vi "SATDdll.vi"(8 "error in (no error)":errorcluster, 11 "SAT Inputs":cluster{"D":dbl, "z":dbl[], "kph":i32}={"D"=0.0, "z"=[0.0, 0.0, 0.0, 0.0, 0.0, 0.0, 0.0, 0.0, 0.0, 0.0, 0.0, 0.0, 0.0, 0.0, 0.0, 0.0, 0.0, 0.0, 0.0, 0.0], "kph"=-1} {"kph" items=["-1 - return middle root (between 0 and 4 C)"=-1, "1 - return highest temperature root (above 4 C)"=1, "3 - return lowest temperature root (along freezing line)"=3]}) -> (0 "error out":errorcluster, 2 "kr":i32(ring)=4 items=["Unknown", "Input state is liquid", "Input state is vapor in equilibrium with liquid", "Input state is liquid in equilibrium with solid (only for pure fluids)", "Input state is vapor in equilibrium with solid (only for pure fluids)", ""], 3 "SAT Outputs":T1={"D"=nan, "e"=nan, "h"=nan, "p"=nan, "s"=nan, "t"=nan, "q"=nan, "Dl"=nan, "Dv"=nan, "x"=[nan, nan, 0.0, 0.0, 0.0, 0.0, 0.0, 0.0, 0.0, 0.0, 0.0, 0.0, 0.0, 0.0, 0.0, 0.0, 0.0, 0.0, 0.0, 0.0], "y"=[nan, nan, 0.0, 0.0, 0.0, 0.0, 0.0, 0.0, 0.0, 0.0, 0.0, 0.0, 0.0, 0.0, 0.0, 0.0, 0.0, 0.0, 0.0, 0.0], "nroot"=0, "k1"=0, "t1"=nan, "p1"=nan, "d1"=nan, "k2"=0, "t2"=nan, "p2"=nan, "d2"=nan, "k3"=0, "t3"=nan, "p3"=nan, "d3"=nan, "ierr"=0, "herr"="", "herr_length"=0})   [LabVIEW 2016]
doc: "subroutine SATD (D,z,kph,kr,t,p,Dl,Dv,x,y,ierr,herr, herr_Length)\n\nIterate for temperature and pressure given a density along the\nsaturation boundary and the composition. \n\n either (Dl,x) or (Dv,y) will correspond to the input state\n with the other pair corresponding to the other phase in equilibrium\n with the input state.\n\nINPUTS:\n D--molar density [mol/L]\n z--composition [array of mol frac]\n kph--flag specifying desired root for multi-valued inputs\n has meaning only for water at temperatures close to its triple point\n -1 = return middle root (between 0 and 4 C)\n 1 = return highest temperature root (above 4 C)\n 3 = return lowest temperature root (along freezing line)\n\nOUTPUTS:\n kr--phase flag: 1 = input state is liquid\n 2 = input state is vapor in equilibrium with liquid\n 3 = input state is liquid in equilibrium with solid (only for pure fluids)\n 4 = input state is vapor in equilibrium with solid (only for pure fluids)\n t--temperature [K]\n p--pressure [kPa]\n Dl--molar density [mol/L] of saturated liquid\n Dv--molar density [mol/L] of saturated vapor\n x--liquid phase composition [array of mol frac]\n y--vapor phase composition [array of mol frac]\n \n ierr--error flag: 0 = successful\n 2 = D > Dmax\n 8 = x out of range\n 10 = D and x out of range\n 160 = CRITP did not converge\n 161 = SATD did not converge\n herr--error string (character*255 variable if ierr<>0)\n herr_length-- length of variable herr (default: 255)"
uses:
  Ctl/SAT_Outputs.ctl
  REFPROP.DLL
panel:
  # "REFPROP-SATDdll.vi"
  # "subroutine SATD (D,z,kph,kr,t,p,Dl,Dv,x,y,ierr,herr, herr_Length)"
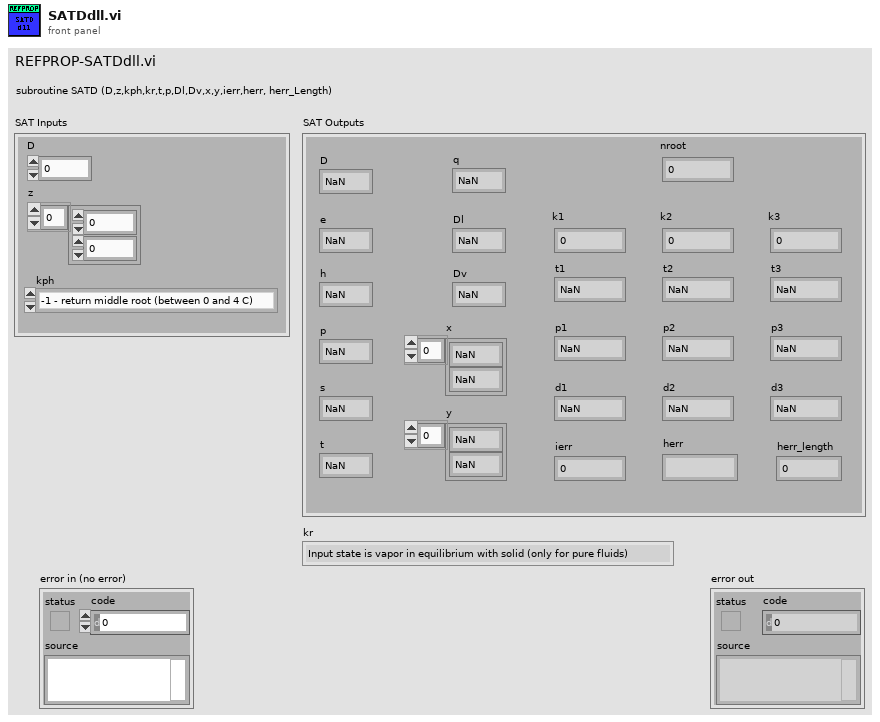
[diagram p1: front panel]
types:
  T1 = typedef "SAT_Outputs.ctl" = cluster{"D":dbl, "e":dbl, "h":dbl, "p":dbl, "s":dbl, "t":dbl, "q":dbl, "Dl":dbl, "Dv":dbl, "x":dbl[], "y":dbl[], "nroot":i32, "k1":i32, "t1":dbl, "p1":dbl, "d1":dbl, "k2":i32, "t2":dbl, "p2":dbl, "d2":dbl, "k3":i32, "t3":dbl, "p3":dbl, "d3":dbl, "ierr":i32, "herr":string, "herr_length":i32}
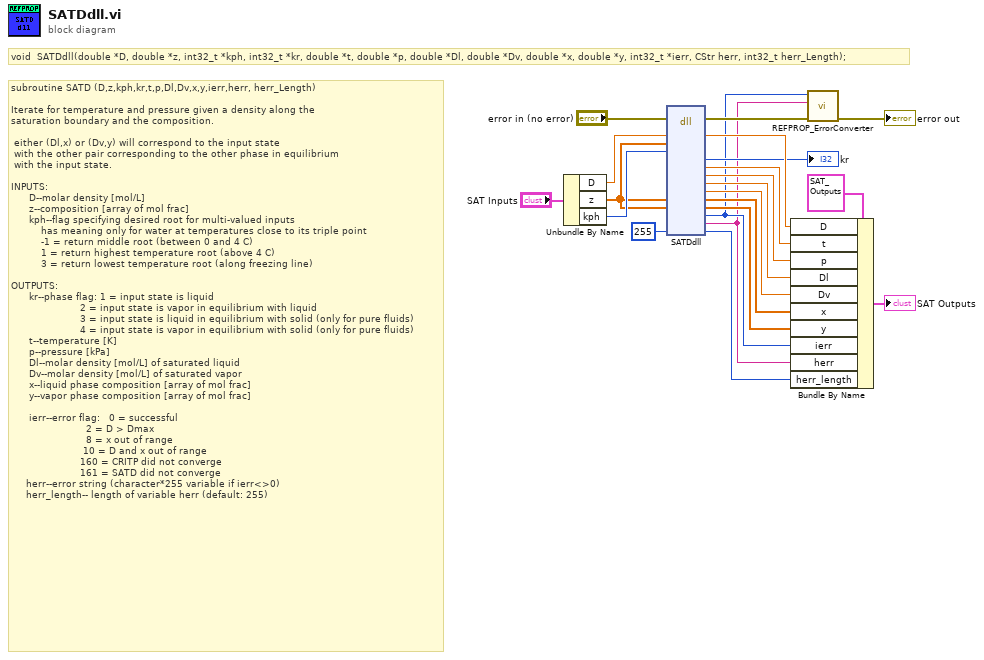
[diagram p0: block diagram]
diagram:
  # "void  SATDdll(double *D, double *z, int32_t *kph, int32_t *kr, double *t, double *p, double *Dl, double *Dv, double *x, double *y, int32_t *ierr, CStr herr, int32_t herr_Length);"
  # "subroutine SATD (D,z,kph,kr,t,p,Dl,Dv,x,y,ierr,herr, herr_Length)\n\nIterate for temperature and pressure given a density along the\nsaturation boundary and the composition. \n\n either (Dl,x) or (Dv,y) will correspond to the input state\n with the other pair corresponding to the other phase in equilibrium\n with the input state.\n\nINPUTS:\n      D--molar density [mol/L]\n      z--composition [array of mol frac]\n      kph--flag specifying desired root for multi-valued inputs\n          has meaning only for water at temperatures close to its triple point\n          -1 = return middle root (between 0 and 4 C)\n          1 = return highest temperature root (above 4 C)\n          3 = return lowest temperature root (along freezing line)\n\nOUTPUTS:\n      kr--phase flag: 1 = input state is liquid\n                       2 = input state is vapor in equilibrium with liquid\n                       3 = input state is liquid in equilibrium with solid (only for pure fluids)\n                       4 = input state is vapor in equilibrium with solid (only for pure fluids)\n      t--temperature [K]\n      p--pressure [kPa]\n      Dl--molar density [mol/L] of saturated liquid\n      Dv--molar density [mol/L] of saturated vapor\n      x--liquid phase composition [array of mol frac]\n      y--vapor phase composition [array of mol frac]\n      \n      ierr--error flag:   0 = successful\n                         2 = D > Dmax\n                         8 = x out of range\n                        10 = D and x out of range\n                       160 = CRITP did not converge\n                       161 = SATD did not converge\n     herr--error string (character*255 variable if ierr<>0)\n     herr_length-- length of variable herr (default: 255)"
  n1 = Unbundle By Name("SAT Inputs") -> ("D"=w17:dbl, "z"=w15:dbl[], "kph"=w16:i32)
  n2 = dll-call lib="C:/Program Files (x86)/REFPROP/REFPROP.*" fn="SATDdll"(error in="error in (no error)", "D"=w17, "z"=w15, "kph"=w16, "x"=w15, "y"=w15, "herr_Length"=255 ("ln")) -> (error out=w19:errorcluster, "D"=w11:dbl, "kr"=→"kr":i32, "t"=w9:dbl, "p"=w8:dbl, "Dl"=w7:dbl, "Dv"=w6:dbl, "x"=w5:dbl[], "y"=w4:dbl[], "ierr"=w3:i32, "herr"=w2:string, "herr_Length"=w1:i32)  [unwired: 12 in, 1 out]
  n3 = Bundle By Name(cluster=T1 {"D"=nan, "e"=nan, "h"=nan, "p"=nan, "s"=nan, "t"=nan, "q"=0.0, "Dl"=nan, "Dv"=nan, "x"=[nan, nan, 0.0, 0.0, 0.0, 0.0, 0.0, 0.0, 0.0, 0.0, 0.0, 0.0, 0.0, 0.0, 0.0, 0.0, 0.0, 0.0, 0.0, 0.0], "y"=[nan, nan, 0.0, 0.0, 0.0, 0.0, 0.0, 0.0, 0.0, 0.0, 0.0, 0.0, 0.0, 0.0, 0.0, 0.0, 0.0, 0.0, 0.0, 0.0], "nroot"=0, "k1"=0, "t1"=nan, "p1"=nan, "d1"=nan, "k2"=0, "t2"=nan, "p2"=nan, "d2"=nan, "k3"=0, "t3"=nan, "p3"=nan, "d3"=nan, "ierr"=0, "herr"="", "herr_length"=0} ("SAT Outputs"), "D"=w11, "t"=w9, "p"=w8, "Dl"=w7, "Dv"=w6, "x"=w5, "y"=w4, "ierr"=w3, "herr"=w2, "herr_length"=w1) -> (→"SAT Outputs":T1)
  n4 = call "REFPROP_ErrorConverter.vi"("error in (no error)"=w19, "Error Message"=w2, "Error Code"=w3) -> ("error out"=→"error out":errorcluster)  [unwired: 8 in]
